vi "Read (Multiple Responses).vi"(8 "error in (no error)":errorcluster, 9 "Wait Time Between Responses (3)":u32=3, 11 "VISA resource name":refnum<visa-resource-name>) -> (0 "error out":errorcluster, 1 "Response Bundle Array":T2(array[cluster]), 2 "Response String Array":string[](array[string]), 3 "VISA resource name out":refnum<visa-resource-name>, 4 "First Response Bundle":T1, 5 "Number of Replies":i32)   [LabVIEW 2018, in "Zaber A Series.lvlib"]
doc: "Reads all available responses from the Serial buffer. An array containing the complete strings of the responses is returned on the Response String Array output, and the details of the format of the response are described here: http://www.zaber.com/wiki/Manuals/ASCII_Protocol_Manual#Replies. This VI also parses the strings, bundles the components, and returns them as an array of bundles on the Response Bundle Array pin. Additionally a pin returns the number of responses received. \n\nThis VI requires that the Initialize VI has been called with the same serial port."
uses:
  Zaber A Series.lvlib
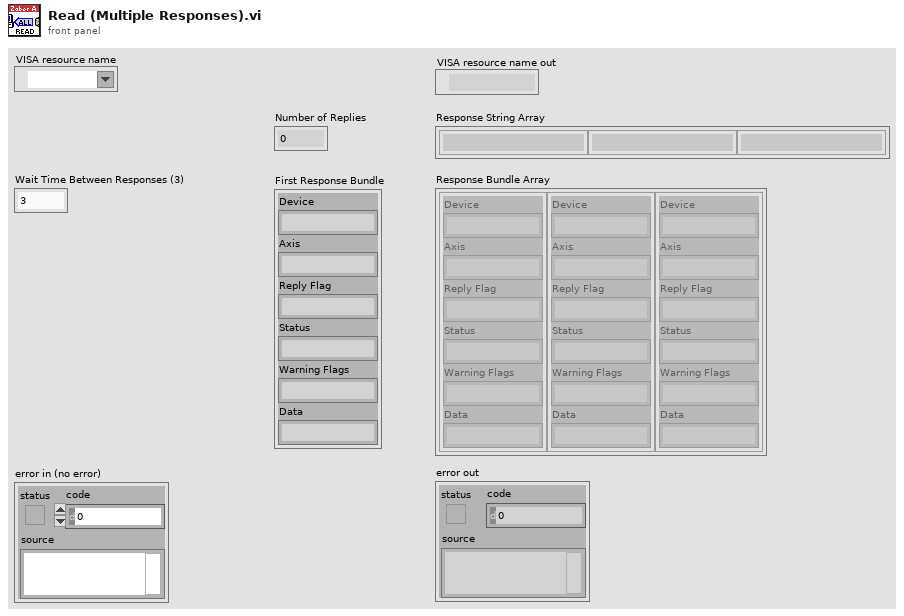
[diagram p1: front panel]
types:
  T1 = cluster{"Device":string, "Axis":string, "Reply Flag":string, "Status":string, "Warning Flags":string, "Data":string}
  T2 = cluster{"Device":string, "Axis":string, "Reply Flag":string, "Status":string, "Warning Flags":string, "Data":string}[]
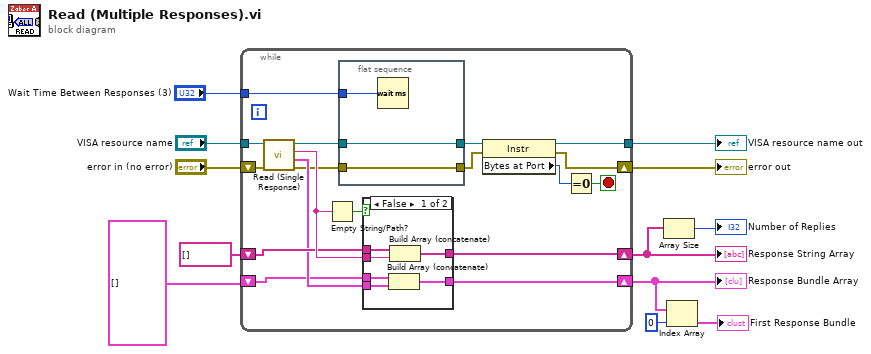
[diagram p0: block diagram]
diagram:
  n1 = while {
    tunnel: "VISA resource name" -> [w30]
    tunnel: [w25] -> w12
    shift-right: [w22] -> w5
    shift-left: string[] [] -> [w21]
    shift-right: [w19] -> w3
    shift-left: T2 [] -> [w18]
    tunnel: "Wait Time Between Responses (3)" -> [w15]
    shift-right: [w28] -> w11
    shift-left: "error in (no error)" -> [w29]
    stop <- w26 stop-if-true
    n2 = call "Read (Single Response).vi"("error in (no error)"=w29, "VISA resource name"=w30) -> ("error out"=w14:errorcluster, "Response Bundle"=w20:T1, "Response"=w23:string, "VISA resource name out"=w17:refnum<visa-resource-name>)  [unwired: 6 in]
    n3 = Empty String/Path?(string/path=w23) -> (empty?=w24:bool)
    n4 = flat-sequence {
      tunnel: w17 -> [w33]
      tunnel: [w33] -> w16
      tunnel: w15 -> [w32]
      tunnel: w14 -> [w31]
      tunnel: [w31] -> w13
      frame #0 {
        n5 = Wait (ms)(milliseconds to wait=w32) -> ()  [unwired: 1 out]
      }
    }
    n6 = case shown="False" w24 {
      tunnel: w23 -> [w39 _]
      tunnel: [w38 w41] -> w22
      tunnel: w21 -> [w37 w41]
      tunnel: w20 -> [w36 _]
      tunnel: [w35 w40] -> w19
      tunnel: w18 -> [w34 w40]
      frame False {
        n7 = Build Array (concatenate)(w34, w36) -> (w35:T2)
        n8 = Build Array (concatenate)(w37, w39) -> (w38:string[])
      }
      frame True {
      }
    }
    n9 = property class="Instr"(reference=w16, error in=w13) -> (reference out=w25:refnum<visa-resource-name>, error out=w28:errorcluster, "Bytes at Port"=w27:u32)
    n10 = Equal To 0?(x=w27) -> (x = 0?=w26:bool)
  }
  "VISA resource name out" <- w12
  "error out" <- w11
  "Response String Array" <- w5
  "Response Bundle Array" <- w3
  n11 = Array Size(array=w5) -> (size(s)=→"Number of Replies":i32)
  n12 = Index Array(array=w3, index=0) -> (element=→"First Response Bundle":T1)
